vi "To String Array.vi"(8 "error in (no error)":errorcluster, 11 "Step Config in":refnum<class "Step Config.lvclass">) -> (0 "error out":errorcluster, 1 "Step String Array":string[](array[string]), 3 "Step Config out":refnum<class "Step Config.lvclass">)   [LabVIEW 2015, in "Step Config.lvclass"]
uses:
  Step Config.lvclass
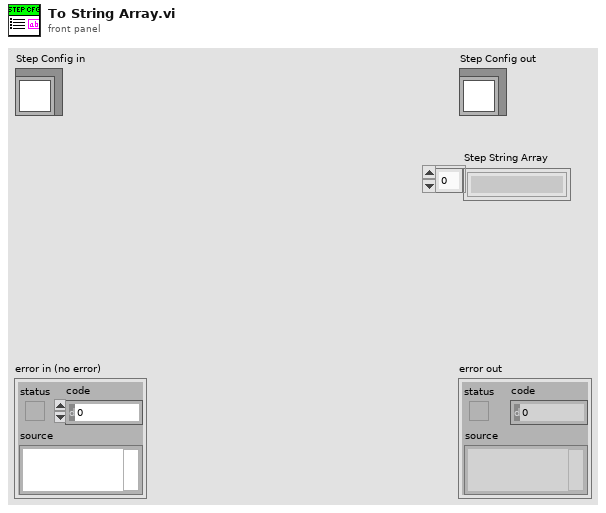
[diagram p1: front panel]
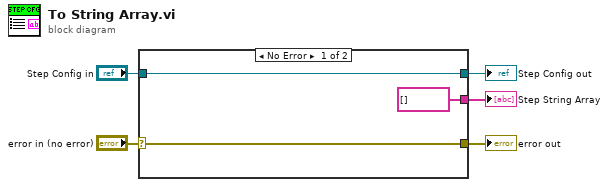
[diagram p0: block diagram]
diagram:
  n1 = case shown="No Error" "error in (no error)" {
    selector: "error in (no error)" -> [w7 w10]
    tunnel: [w7 w10] -> w4
    tunnel: [w8 w9] -> w2
    tunnel: "Step Config in" -> [w8 w9]
    tunnel: [string[] [] ("Array") _] -> w1
    frame No Error {
    }
    frame Error {
    }
  }
  "error out" <- w4
  "Step Config out" <- w2
  "Step String Array" <- w1
